vi "Initialize Sink.vi"(11 "String Control Sink in":refnum<class "String Control Sink.lvclass">) -> (0 "error out":errorcluster, 3 "String Control Sink out":refnum<class "String Control Sink.lvclass">)   [LabVIEW 2018, in "MVA Framework.lvlib" / "String Control Sink.lvclass"]
uses:
  String Control Sink.lvclass
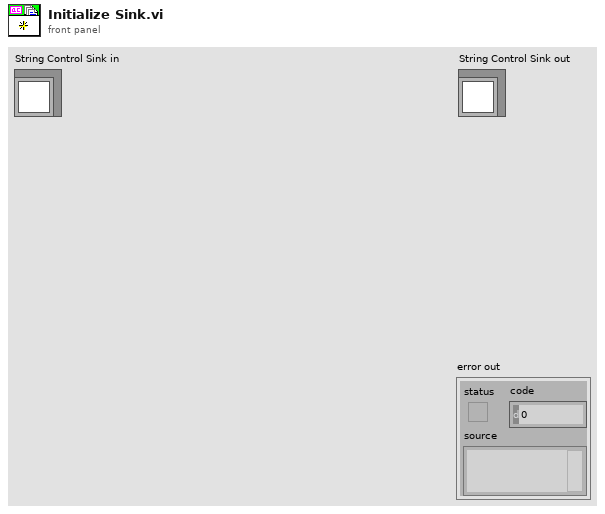
[diagram p1: front panel]
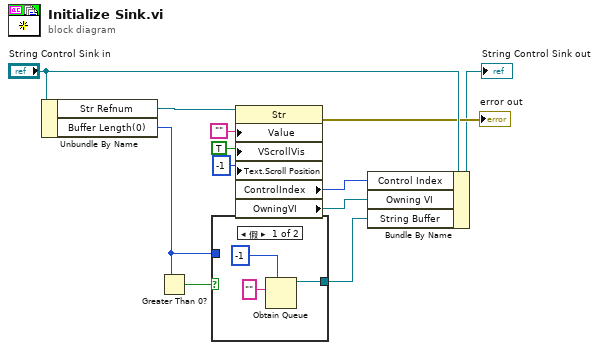
[diagram p0: block diagram]
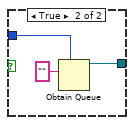
[diagram p2: hidden frame]
diagram:
  n1 = Unbundle By Name("String Control Sink in") -> ("Str Refnum"=w12:refnum<vi>, "Buffer Length(0)"=w1:u32)
  n2 = Greater Than 0?(x=w1) -> (x > 0?=w2:bool)
  n3 = case shown="假" w2 {
    tunnel: w1 -> [_ w17]
    tunnel: [w14 w16] -> w3
    frame False {
      n4 = Obtain Queue(max queue size (-1, unlimited)=-1, element data type="") -> (queue out=w14:refnum<queue>)  [unwired: 3 in, 2 out]
    }
    frame True {
      n5 = Obtain Queue(max queue size (-1, unlimited)=w17, element data type="") -> (queue out=w16:refnum<queue>)  [unwired: 3 in, 2 out]
    }
  }
  n6 = property class="Str"(reference=w12, "Value"="", "VScrollVis"=TRUE ("Vertical Scrollbar Visible"), "Text.Scroll Position"=-1) -> (error out=→"error out":errorcluster, "ControlIndex"=w5:i32, "OwningVI"=w4:refnum<vi>)  [unwired: 1 in, 1 out]
  n7 = Bundle By Name(cluster="String Control Sink in", "Control Index"=w5, "Owning VI"=w4, "String Buffer"=w3) -> (→"String Control Sink out":refnum<class "String Control Sink.lvclass">)
